vi "readU32FIFO.vi"(8 "error in (no error)":errorcluster, 9 "Timeout":i32, 10 "NumberOfElements":u32, 11 "IReadU32FIFO in":refnum<class "IReadU32FIFO.lvclass">) -> (0 "error out":errorcluster, 1 "ElementsRemaining":u32, 2 "Data":u32[](array[numeric]), 3 "IReadU32FIFO out":refnum<class "IReadU32FIFO.lvclass">)   [LabVIEW 2015, in "RTFPGA.lvlib" / "IReadU32FIFO.lvclass"]
uses:
  IReadU32FIFO.lvclass
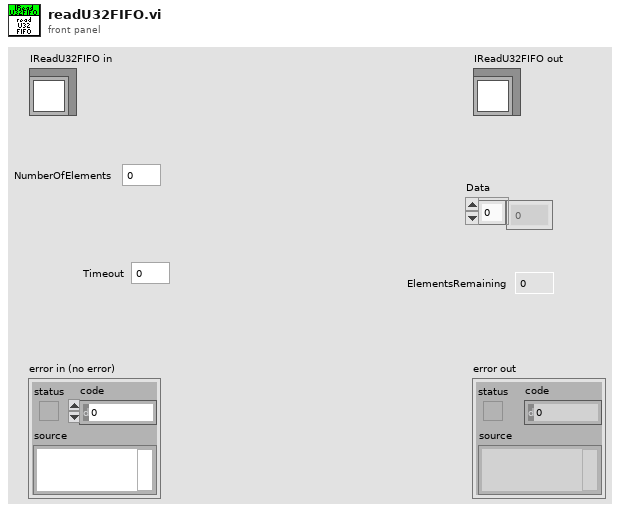
[diagram p1: front panel]
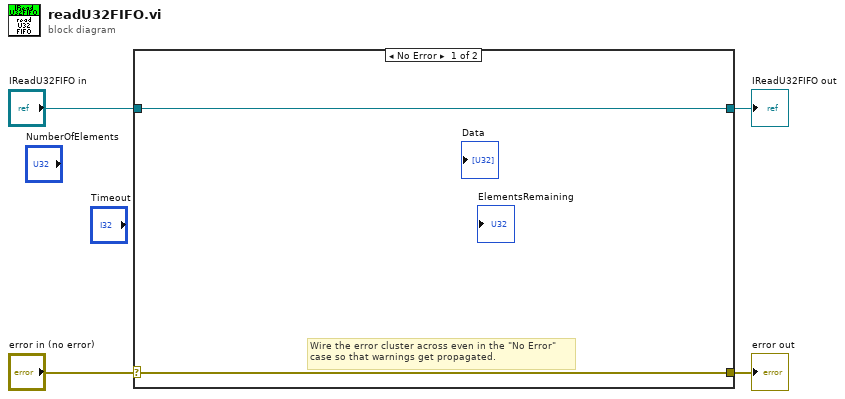
[diagram p0: block diagram]
diagram:
  n1 = case shown="No Error" "error in (no error)" {
    selector: "error in (no error)" -> [w5 w8]
    tunnel: [w5 w8] -> w3
    tunnel: [w6 w7] -> w1
    tunnel: "IReadU32FIFO in" -> [w6 w7]
    frame No Error {
      # "Wire the error cluster across even in the \"No Error\"\ncase so that warnings get propagated."
    }
    frame Error {
    }
  }
  "error out" <- w3
  "IReadU32FIFO out" <- w1
